vi "test_Util_AprilTagUtils.vi"(8 "error in (no error)":errorcluster) -> (0 "error out":errorcluster, 3 "Test Passed":bool)   [LabVIEW 2019]
uses:
  <vilib>/Rock Robotics/WPI/ThirdParty/JAS_Junk/TrajLib/TypeDef/POSE3D.ctl
  <vilib>/Rock Robotics/WPI/ThirdParty/JAS_Junk/TrajLib/TypeDef/TRANSLATION3D.ctl
  <vilib>/Rock Robotics/WPI/ThirdParty/JAS_Junk/TrajLib/TypeDef/ROTATION3D.ctl
  <vilib>/Rock Robotics/WPI/ThirdParty/JAS_Junk/TrajLib/TypeDef/QUATERNION.ctl
  <vilib>/Rock Robotics/WPI/ThirdParty/JAS_Junk/TrajLib/VI/Translation3d_Create_Default.vi
  <vilib>/Rock Robotics/WPI/ThirdParty/JAS_Junk/TrajLib/VI/Quaternion_New_Default.vi
  <vilib>/Rock Robotics/WPI/ThirdParty/JAS_Junk/TrajLib/Conv_Deg_Radians.vi
  <vilib>/Rock Robotics/WPI/ThirdParty/JAS_Junk/TrajLib/Rotation2d_CreateAngle.vi
  <vilib>/Rock Robotics/WPI/ThirdParty/JAS_Junk/TrajLib/Pose2d_getTranslation.vi
  <vilib>/Rock Robotics/WPI/ThirdParty/JAS_Junk/TrajLib/Pose2d_RelativeTo.vi
  <vilib>/Rock Robotics/WPI/ThirdParty/JAS_Junk/TrajLib/Translation2d_GetXY.vi
  <vilib>/Rock Robotics/WPI/ThirdParty/JAS_Junk/TrajLib/Rotation2d_CreateXY.vi
  <vilib>/Rock Robotics/WPI/ThirdParty/JAS_Junk/TrajLib/Rotation2d_GetRadians.vi
  <vilib>/Rock Robotics/WPI/ThirdParty/JAS_Junk/TrajLib/VI/Quaternion_New.vi
  <vilib>/Rock Robotics/WPI/ThirdParty/JAS_Junk/TrajLib/VI/Pose3d_New_Trans3dRot3d.vi
  <vilib>/Rock Robotics/WPI/ThirdParty/JAS_Junk/TrajLib/VI/Pose3d_Plus.vi
  <vilib>/Rock Robotics/WPI/ThirdParty/JAS_Junk/TrajLib/VI/Transform3d_Inverse.vi
  <vilib>/Rock Robotics/WPI/ThirdParty/JAS_Junk/TrajLib/VI/Pose3d_getTranslation3d.vi
  <vilib>/Rock Robotics/WPI/ThirdParty/JAS_Junk/TrajLib/VI/Translation3d_GetXYZ.vi
  <vilib>/Rock Robotics/WPI/ThirdParty/JAS_Junk/TrajLib/Transform2d_Create_PosePose.vi
  <vilib>/Rock Robotics/WPI/ThirdParty/JAS_Junk/TrajLib/Util_CalcDist.vi
  <vilib>/Rock Robotics/WPI/ThirdParty/JAS_Junk/TrajLib/VI/Pose3d_TransformBy.vi
  <vilib>/Rock Robotics/WPI/ThirdParty/JAS_Junk/TrajLib/VI/Rotation3d_UnaryMinus.vi
  <vilib>/Rock Robotics/WPI/ThirdParty/JAS_Junk/TrajLib/VI/Translation3d_RotateBy.vi
  <vilib>/Rock Robotics/WPI/ThirdParty/JAS_Junk/TrajLib/VI/Translation3d_UnaryMinus.vi
  <vilib>/Rock Robotics/WPI/ThirdParty/JAS_Junk/TrajLib/VI/Transform3d_GetTranslation3d.vi
  <vilib>/Rock Robotics/WPI/ThirdParty/JAS_Junk/TrajLib/VI/Transform3d_GetRotation3d.vi
  <vilib>/Rock Robotics/WPI/ThirdParty/JAS_Junk/TrajLib/Rotation2d_UnaryMinus.vi
  <vilib>/Rock Robotics/WPI/ThirdParty/JAS_Junk/TrajLib/Translation2d_RotateBy.vi
  <vilib>/Rock Robotics/WPI/ThirdParty/JAS_Junk/TrajLib/Translation2d_Minus.vi
  <vilib>/Rock Robotics/WPI/ThirdParty/JAS_Junk/TrajLib/Rotation2d_Minus.vi
  <vilib>/Rock Robotics/WPI/ThirdParty/JAS_Junk/TrajLib/VI/Pose3d_getRotation3d.vi
  <vilib>/Rock Robotics/WPI/ThirdParty/JAS_Junk/TrajLib/VI/Translation3d_Plus.vi
  <vilib>/Rock Robotics/WPI/ThirdParty/JAS_Junk/TrajLib/VI/Rotation3d_Plus.vi
  <vilib>/Rock Robotics/WPI/ThirdParty/JAS_Junk/TrajLib/VI/Rotation3d_Create_Quaternion.vi
  <vilib>/Rock Robotics/WPI/ThirdParty/JAS_Junk/TrajLib/VI/Quaternion_Inverse.vi
  <vilib>/Rock Robotics/WPI/ThirdParty/JAS_Junk/TrajLib/VI/Rotation3d_GetQuaterion.vi
  <vilib>/Rock Robotics/WPI/ThirdParty/JAS_Junk/TrajLib/VI/Quaternion_Times.vi
  <vilib>/Rock Robotics/WPI/ThirdParty/JAS_Junk/TrajLib/VI/Quaternion_Get_All.vi
  <vilib>/Rock Robotics/WPI/ThirdParty/JAS_Junk/TrajLib/Rotation2d_RotateBy.vi
  <vilib>/Rock Robotics/WPI/ThirdParty/JAS_Junk/TrajLib/VI/Rotation3d_RotateBy.vi
  <vilib>/Rock Robotics/WPI/ThirdParty/JAS_Junk/TrajLib/VI/Quaternion_Normalize.vi
  <vilib>/Rock Robotics/WPI/ThirdParty/JAS_Junk/TrajLib/Trajectory_Library.lvlib
  PhotonVisionLib/PhotonVisionLib.lvlib
panel:
  out "FieldToRpbotPose3d":T1={"Translation3d"={"X"=0.0, "Y"=0.0, "Z"=0.0}, "Rotation3d"={"Q_quaternion"={"R"=1.0, "V"=[0.0, 0.0, 0.0]}}} {"Translation3d"."Z" format="%14.3f"; "Translation3d"."Y" format="%14.3f"; "Translation3d"."X" format="%14.3f"}
  out "Test 1 Passed":bool
  out "Test 0 Passed":bool
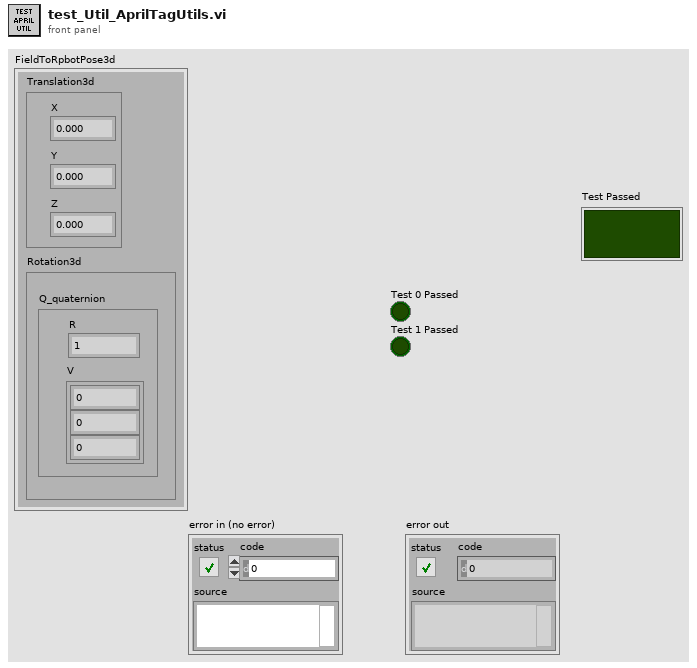
[diagram p1: front panel]
types:
  T1 = typedef "Trajectory_Library.lvlib/POSE3D.ctl" = cluster{"Translation3d":T2, "Rotation3d":T3}
  T2 = typedef "Trajectory_Library.lvlib/TRANSLATION3D.ctl" = cluster{"X":dbl, "Y":dbl, "Z":dbl}
  T3 = typedef "Trajectory_Library.lvlib/ROTATION3D.ctl" = cluster{"Q_quaternion":T4}
  T4 = typedef "Trajectory_Library.lvlib/QUATERNION.ctl" = cluster{"R":dbl, "V":dbl[]}
  T5 = typedef "Trajectory_Library.lvlib/TRANSFORM3D.ctl" = cluster{"TRANSLATION3D":T2, "ROTATION3D":T3, "XF":bool}
  T6 = typedef "Trajectory_Library.lvlib/ROTATION2D.ctl" = cluster{"VALUE":dbl, "COS":dbl, "SIN":dbl}
  T7 = typedef "Trajectory_Library.lvlib/TRANSLATION2D.ctl" = cluster{"X":dbl, "Y":dbl}
  T8 = typedef "Trajectory_Library.lvlib/POSE2D.ctl" = cluster{"TRANSLATION":T7, "ROTATION":T6}
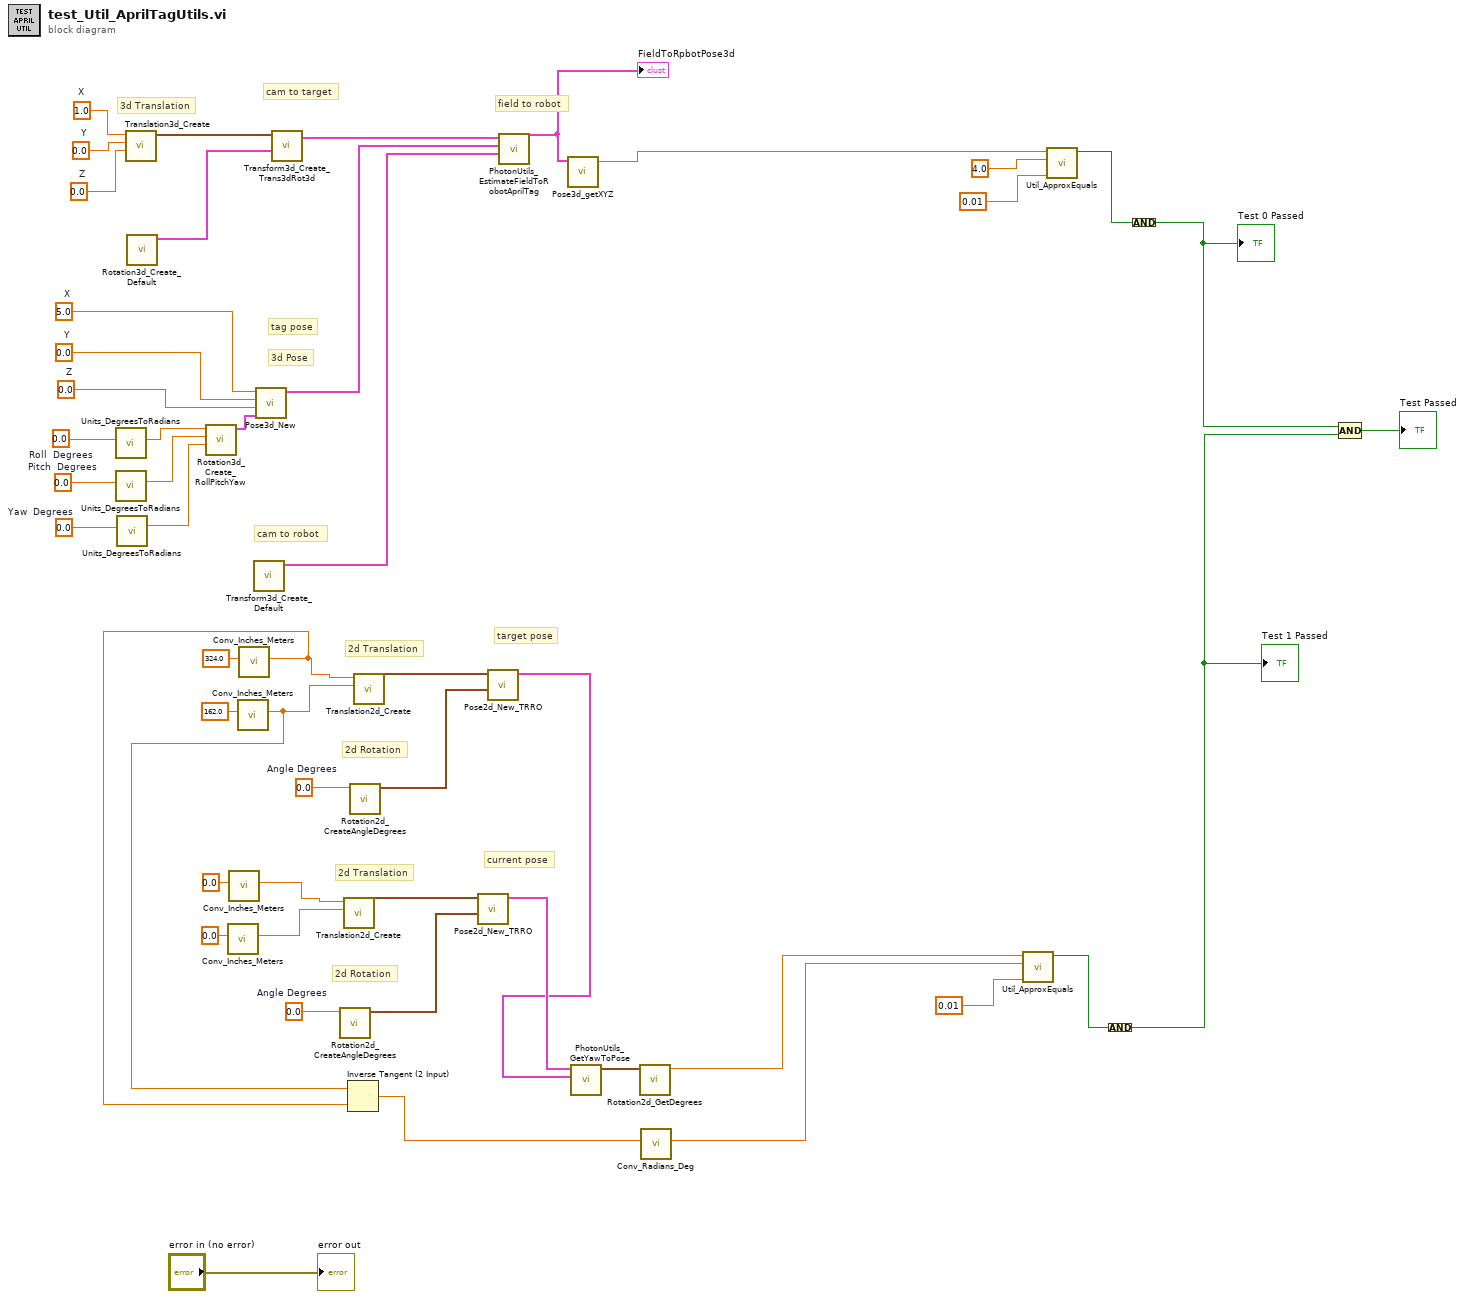
[diagram p0: block diagram]
diagram:
  w13 = 0.0  # Angle Degrees
  w18 = 0.0  # Angle Degrees
  w34 = 5.0  # X
  w33 = 0.0  # Y
  w32 = 0.0  # Z
  w26 = 0.0  # Roll  Degrees
  w27 = 0.0  # Pitch  Degrees
  w28 = 0.0  # Yaw  Degrees
  w40 = 0.0  # Z
  w39 = 1.0  # X
  w38 = 0.0  # Y
  # "current pose"
  # "2d Rotation"
  # "2d Translation"
  # "target pose"
  # "2d Rotation"
  # "2d Translation"
  # "field to robot"
  # "cam to robot"
  # "tag pose"
  # "cam to target"
  # "3d Pose"
  # "3d Translation"
  n1 = call <vilib>:"Units_DegreesToRadians.vi"("Degrees"=w26) -> ("Radians"=w29:dbl)  [unwired: 10 in]
  n2 = call <vilib>:"Units_DegreesToRadians.vi"("Degrees"=w27) -> ("Radians"=w30:dbl)  [unwired: 10 in]
  n3 = call <vilib>:"Units_DegreesToRadians.vi"("Degrees"=w28) -> ("Radians"=w31:dbl)  [unwired: 10 in]
  n4 = call <vilib>:"Translation3d_Create.vi"("Z"=w40, "Y"=w38, "X"=w39) -> ("TRANSLATION3D"=w37:T2)  [unwired: 8 in]
  n5 = call <vilib>:"Rotation3d_Create_Default.vi"() -> ("ROTATION3D"=w36:T3)  [unwired: 11 in]
  n6 = call <vilib>:"Rotation3d_Create_RollPitchYaw.vi"("Yaw"=w31, "Pitch"=w30, "Roll"=w29) -> ("Rotation3d"=w35:T3)  [unwired: 8 in]
  n7 = call <vilib>:"Conv_Inches_Meters.vi"("INCH"=0.0) -> ("Meters"=w11:dbl)  [unwired: 10 in]
  n8 = call <vilib>:"Conv_Inches_Meters.vi"("INCH"=0.0) -> ("Meters"=w12:dbl)  [unwired: 10 in]
  n9 = call <vilib>:"Conv_Inches_Meters.vi"("INCH"=162.0) -> ("Meters"=w8:dbl)  [unwired: 10 in]
  n10 = call <vilib>:"Conv_Inches_Meters.vi"("INCH"=324.0) -> ("Meters"=w7:dbl)  [unwired: 10 in]
  n11 = call <vilib>:"Transform3d_Create_Default.vi"() -> ("Transform3d"=w23:T5)  [unwired: 11 in]
  n12 = call <vilib>:"Pose3d_New.vi"("Rotation3d"=w35, "z"=w32, "Y"=w33, "X"=w34) -> ("out Pose3d"=w24:T1)  [unwired: 7 in]
  n13 = call <vilib>:"Transform3d_Create_Trans3dRot3d.vi"("Rotation3d"=w36, "Translation3d"=w37) -> ("Transform3d"=w25:T5)  [unwired: 9 in]
  n14 = call <vilib>:"Rotation2d_CreateAngleDegrees.vi"("Angle_Degrees"=w13) -> ("ROTATION"=w9:T6)  [unwired: 10 in]
  n15 = call <vilib>:"Translation2d_Create.vi"("Y"=w11, "X"=w12) -> ("TRANSLATION"=w10:T7)  [unwired: 9 in]
  n16 = Inverse Tangent (2 Input)(1:w7, 2:w8) -> (0:w3:dbl)
  n17 = call <vilib>:"Rotation2d_CreateAngleDegrees.vi"("Angle_Degrees"=w18) -> ("ROTATION"=w16:T6)  [unwired: 10 in]
  n18 = call <vilib>:"Translation2d_Create.vi"("Y"=w8, "X"=w7) -> ("TRANSLATION"=w17:T7)  [unwired: 9 in]
  n19 = call <vilib>:"Pose2d_New_TRRO.vi"("ROTATION"=w9, "TRANSLATION"=w10) -> ("outPOSE"=w2:T8)  [unwired: 9 in]
  n20 = call <vilib>:"Pose2d_New_TRRO.vi"("ROTATION"=w16, "TRANSLATION"=w17) -> ("outPOSE"=w1:T8)  [unwired: 9 in]
  n21 = call "PhotonUtils_EstimateFieldToRobotAprilTag.vi"("CameraToRobotTransform3d"=w23, "FieldRelativeTagPose3d"=w24, "CameraToTargetTransform3d"=w25) -> ("FieldToRpbotPose3d"=w21:T1)  [unwired: 8 in]
  "FieldToRpbotPose3d" <- w21
  n22 = call <vilib>:"Pose3d_getXYZ.vi"("in Pose3d"=w21) -> ("X"=w22:dbl)  [unwired: 8 in, 2 out]
  n23 = call "PhotonUtils_GetYawToPose.vi"("TargetPose"=w1, "RobotPose"=w2) -> ("YawToPose"=w6:T6)  [unwired: 9 in]
  n24 = call <vilib>:"Rotation2d_GetDegrees.vi"("in ROTATION"=w6) -> ("AngleDegrees"=w5:dbl)  [unwired: 10 in]
  n25 = call <vilib>:"Conv_Radians_Deg.vi"("Radians"=w3) -> ("Degrees"=w4:dbl)  [unwired: 10 in]
  n26 = call <vilib>:"Util_ApproxEquals.vi"("Tolerance"=0.01, "Value 2"=w4, "Value 1"=w5) -> ("ApproxEquals"=w44:bool)  [unwired: 8 in]
  n27 = call <vilib>:"Util_ApproxEquals.vi"("Tolerance"=0.01, "Value 2"=4.0, "Value 1"=w22) -> ("ApproxEquals"=w45:bool)  [unwired: 8 in]
  n28 = Compound Arithmetic op=AND(w44) -> (w41:bool)
  "Test 1 Passed" <- w41
  n29 = Compound Arithmetic op=AND(w45) -> (w42:bool)
  "Test 0 Passed" <- w42
  n30 = Compound Arithmetic op=AND(w42, w41) -> (→"Test Passed":bool)
  "error out" <- "error in (no error)"
